vi "circle.vi"() -> ()   [LabVIEW 2018]
panel:
  out "XY Graph":cluster{dbl[], dbl[]}(graph)
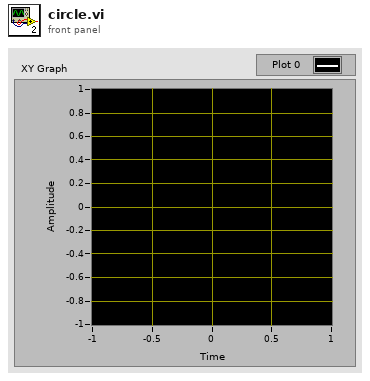
[diagram p1: front panel]
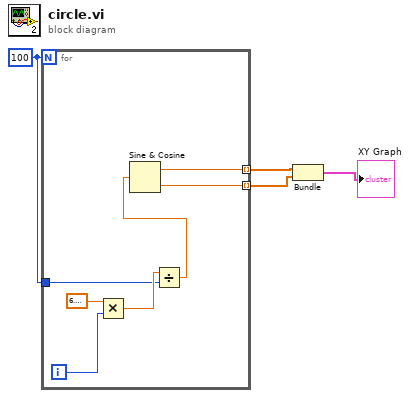
[diagram p0: block diagram]
diagram:
  w4 = 100
  n1 = for {
    N: w4 -> [_]
    tunnel: w4 -> [w9]
    tunnel: [w6] -> w3 mode=indexing
    tunnel: [w5] -> w2 mode=indexing
    i -> [w11]
    n2 = Multiply(x=6.283185307179586, y=w11) -> (x*y=w10:dbl)
    n3 = Divide(x=w10, y=w9) -> (x/y=w8:dbl)
    n4 = Sine & Cosine(0:w8) -> (1:w6:dbl, 2:w5:dbl)
  }
  n5 = Bundle(w3, w2) -> (→"XY Graph":cluster{dbl[], dbl[]})  [unwired: 1 in]
